vi "PrepLine_window.vi"() -> ()   [LabVIEW 2015]
uses:
  <vilib>/Utility/miscctls.llb/LVPoint32TypeDef.ctl
  global variables.vi
  Classes/StatusLog/StatusLog.lvclass
  Classes/PrepLineObject/PrepLineObject.lvclass
panel:
  out "name of changed":string
  out "Button":u16
  out "Mouse Down \nCoords":T1
  in  "error in (no error)":errorcluster
  out "prepline picture":picture
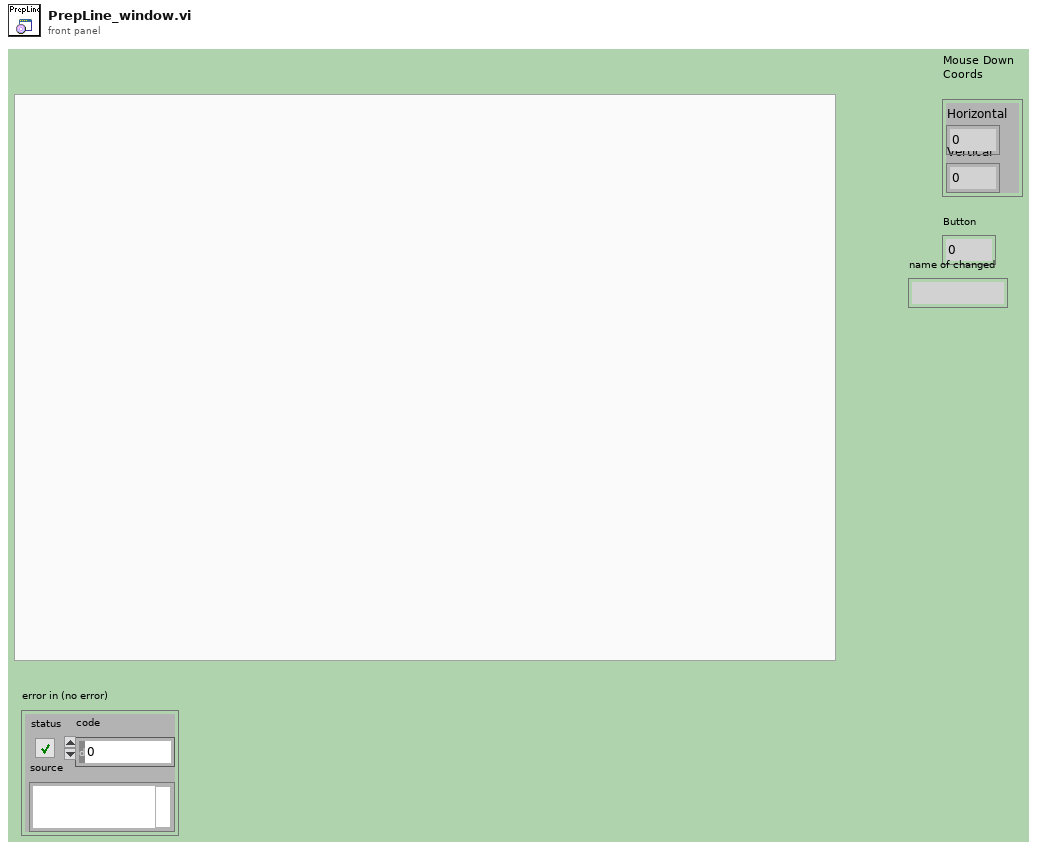
[diagram p1: front panel]
types:
  T1 = typedef "LVPoint32TypeDef.ctl" = cluster{"Horizontal":i32, "Vertical":i32}
  T2 = typedef "LVRectTypeDef.ctl" = cluster{"Left":i16, "Top":i16, "Right":i16, "Bottom":i16}
  T3 = typedef "imagedata.ctl" = cluster{"image type":i32, "image depth":i32, "image":u8[], "mask":u8[], "colors":u32[], "Rectangle":cluster{"left":i16, "top":i16, "right":i16, "bottom":i16}}
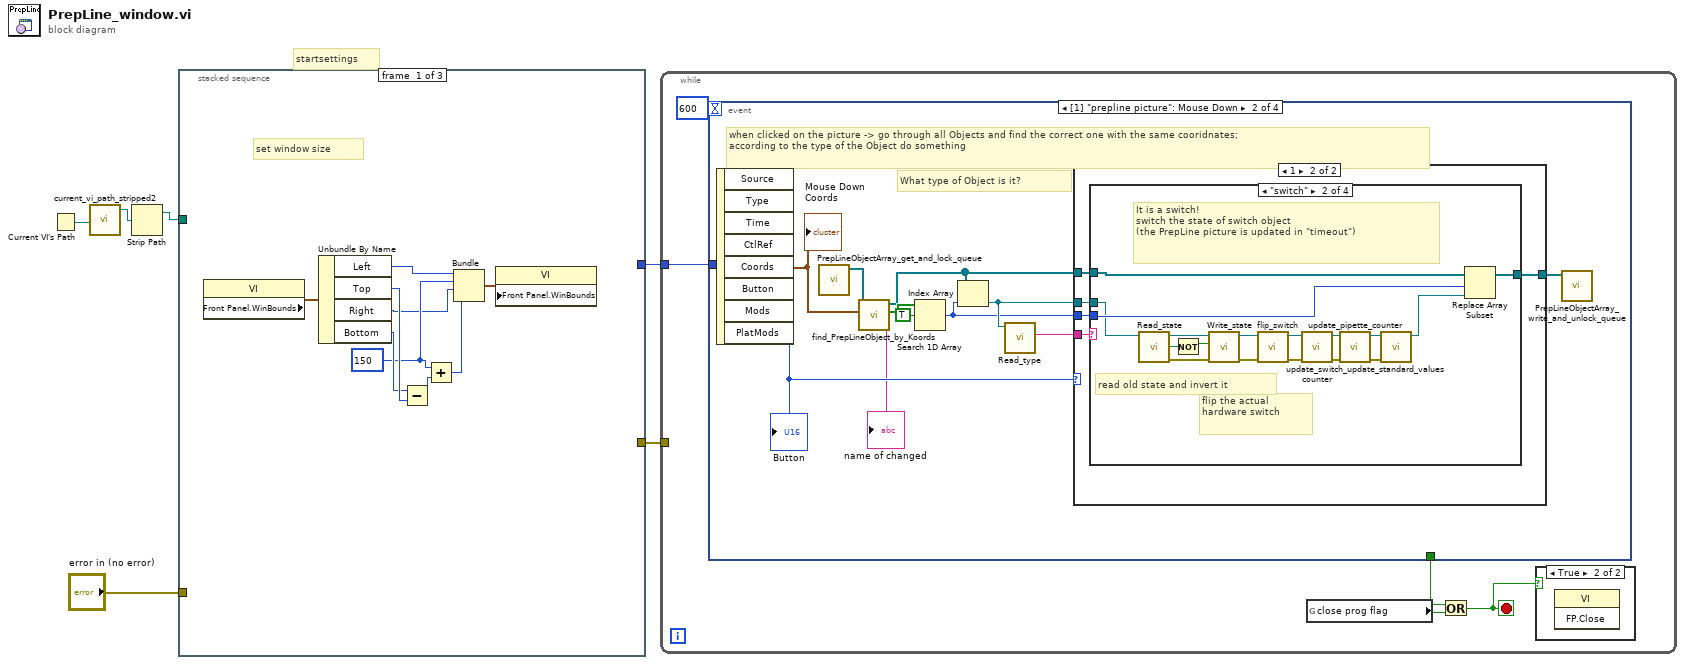
[diagram p0: block diagram]
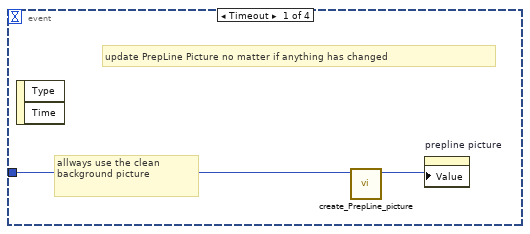
[diagram p3: hidden frame]
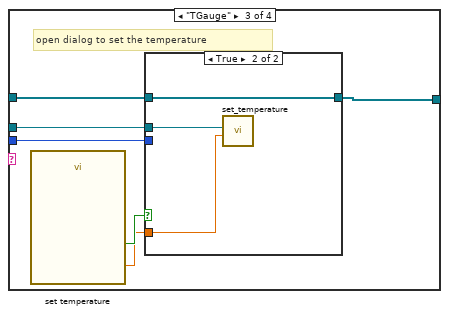
[diagram p6: hidden frame]
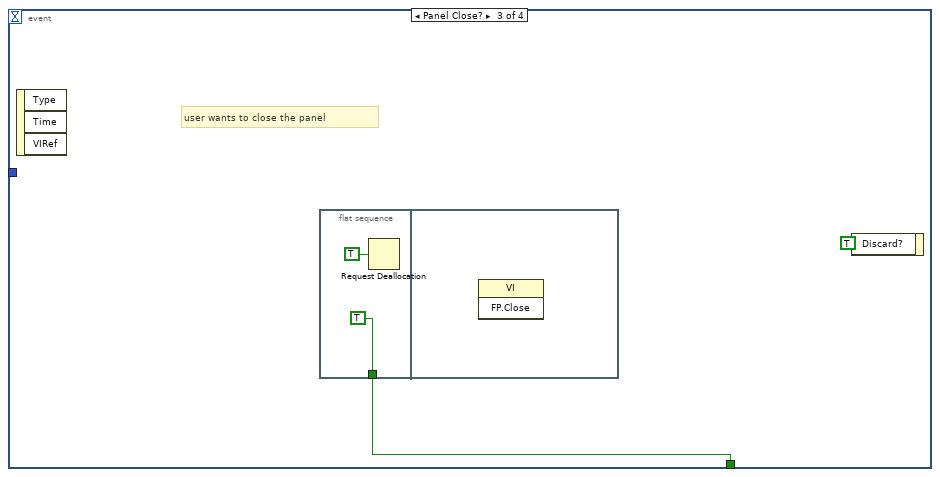
[diagram p9: hidden frame]
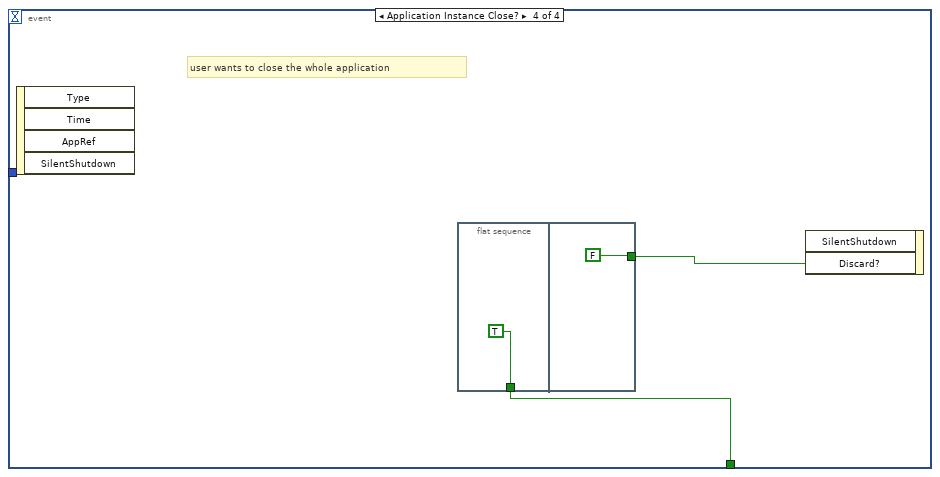
[diagram p10: hidden frame]
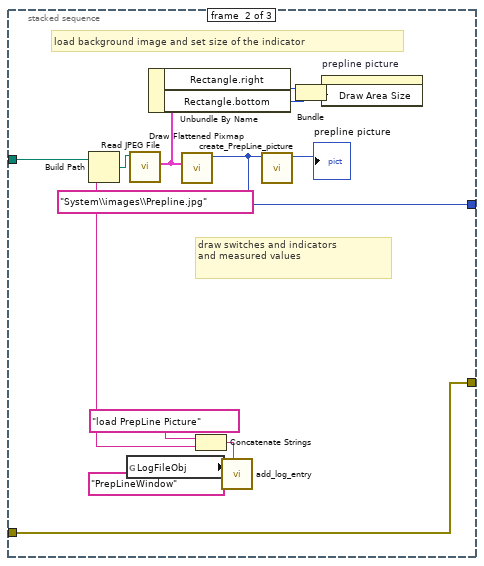
[diagram p11: hidden frame]
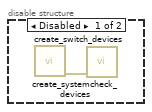
[diagram p13: hidden frame]
diagram:
  # "startsettings"
  n1 = Current VI's Path() -> (path=w3:path)
  n2 = call "current_vi_path_stripped2.vi"("current VI Path"=w3) -> ("current VI Path stripped out"=w1:path)  [unwired: 3 in, 1 out]
  n3 = Strip Path(path=w1) -> (stripped path=w2:path)  [unwired: 1 out]
  n4 = stacked-sequence {
    tunnel: [_ w28 _] -> w6
    tunnel: w2 -> [_ w29 _]
    tunnel: "error in (no error)" -> [_ w28 _]
    tunnel: [_ w16 _] -> w4
    frame #0 {
      w11 = i16 150 ("y")
      # "set window size"
      n5 = property class="VI"() -> ("Front Panel.WinBounds"=w7:T2)  [unwired: 2 in, 2 out]
      n6 = Unbundle By Name(w7) -> ("Left"=w8:i16, "Top"=w15:i16, "Right"=w10:i16, "Bottom"=w14:i16)
      n7 = Subtract(x=w14, y=w15) -> (x-y=w12:i16)
      n8 = Add(x=w11, y=w12) -> (x+y=w13:i16)
      n9 = Bundle("Left"=w8, "y"=w11, "Right"=w10, w13) -> (w9:cluster{"Left":i16, "y":i16, "Right":i16, i16})  [unwired: 1 in]
      n10 = property class="VI"("Front Panel.WinBounds"=w9) -> ()  [unwired: 2 in, 2 out]
    }
    frame #1 {
      w18 = "System\\images\\Prepline.jpg" ("name or relative path")
      # "draw switches and indicators\nand measured values"
      # "load background image and set size of the indicator"
      n11 = Build Path(base path=w29, name or relative path=w18) -> (appended path=w20:path)
      n12 = global read "global variables.vi" "LogFileObj"() -> (w23:refnum<class "StatusLog.lvclass">)
      n13 = call <vilib>:"Read JPEG File.vi"("path to JPEG file"=w20) -> ("image data"=w27:T3)  [unwired: 8 in, 2 out]
      n14 = Unbundle By Name(w27) -> ("Rectangle.right"=w26:i16, "Rectangle.bottom"=w25:i16)
      n15 = call <vilib>:"Draw Flattened Pixmap.vi"("image data"=w27) -> ("new picture"=w16:picture)  [unwired: 8 in]
      n16 = Concatenate Strings("load PrepLine Picture" ("new entry"), w18) -> (w21:string)
      n17 = call-dynamic "add_log_entry.vi"("new entry"=w21, "log identifiers"="PrepLineWindow", "StatusLog in"=w23) -> ()  [unwired: 5 in, 2 out]
      n18 = call "create_PrepLine_picture.vi"("Value in"=w16) -> ("Value out"=→"prepline picture":picture)  [unwired: 10 in]
      n19 = Bundle("right"=w26, "bottom"=w25) -> (w24:cluster{"right":i16, "bottom":i16})  [unwired: 1 in]
      n20 = property on="prepline picture" class="Pict"("Draw Area Size"=w24) -> ()  [unwired: 2 in, 2 out]
    }
    frame #2 {
      # "this is usually done in the main vi of the\nprogram and not here; use thos only\nfor test purposes"
      # "read switch preferences out of switch file\nand generate switch objects - stored together with all\nother objects  in global variable"
      n21 = disable-structure shown="Enabled" {
        frame Disabled {
          n22 = call "create_switch_devices.vi"() -> ("error out"=w30:errorcluster)  [unwired: 11 in]
          n23 = call "create_systemcheck_devices.vi"("error in (no error)"=w30) -> ()  [unwired: 10 in, 1 out]
        }
        frame Enabled {
        }
      }
    }
  }
  n24 = while {
    tunnel: w6 -> [_]
    tunnel: w4 -> [w34]
    stop <- w31 stop-if-true
    n25 = event shown="[1] \"prepline picture\": Mouse Down" {
      selector: _ -> [_ _ _ _]
      dyn-events: _ -> [_ _ _ _]
      timeout: 600 -> [_ _ _ _]
      tunnel: [_ _ w85 w89] -> w33
      tunnel: w34 -> [w36 _ _ _]
      event Timeout {
        # "allways use the clean\nbackground picture"
        # "update PrepLine Picture no matter if anything has changed"
        n26 = event-data() -> ()  [unwired: 1 in, 2 out]
        n27 = call "create_PrepLine_picture.vi"("Value in"=w36) -> ("Value out"=w37:picture)  [unwired: 10 in]
        n28 = property on="prepline picture" class="Pict"("Value"=w37) -> ()  [unwired: 2 in, 2 out]
      }
      event "prepline picture": Mouse Down {
        # "What type of Object is it?"
        # "when clicked on the picture -> go through all Objects and find the correct one with the same cooridnates;\naccording to the type of the Object do something"
        n29 = event-data() -> ("Coords"=w41:T1, "Button"=w44:u16)  [unwired: 1 in, 6 out]
        "Mouse Down \nCoords" <- w41
        "Button" <- w44
        n30 = call "PrepLineObjectArray_get_and_lock_queue.vi"() -> ("PrepLineObjects"=w39:refnum<class "PrepLineObject.lvclass">[])  [unwired: 10 in, 1 out]
        n31 = call "find_PrepLineObject_by_Koords.vi"("Coords"=w41, "PrepLine\nobjects in"=w39) -> ("name of changed"=→"name of changed":string, "changed switch array"=w48:bool[], "PrepLineObjectsOut"=w40:refnum<class "PrepLineObject.lvclass">[])  [unwired: 5 in, 1 out]
        n32 = Search 1D Array(1D array=w48, element=TRUE) -> (index of element=w43:i32)  [unwired: 1 in]
        n33 = Index Array(array=w40, index=w43) -> (element=w46:refnum<class "PrepLineObject.lvclass">)
        n34 = call-dynamic "Read_type.vi"("PrepLinePictureObjects in"=w46) -> ("type"=w45:string)  [unwired: 8 in, 2 out]
        n35 = case shown="1" w44 {
          tunnel: w40 -> [w49 w54]
          tunnel: w43 -> [_ w53]
          tunnel: w46 -> [_ w52]
          tunnel: w45 -> [_ w51]
          tunnel: [w49 w50] -> w38
          frame 0, Default {
          }
          frame 1 {
            n36 = case shown="\"switch\"" w51 {
              tunnel: w54 -> [w55 w72 w76 w83]
              tunnel: w53 -> [_ w71 w74 _]
              tunnel: w52 -> [_ w63 w75 _]
              tunnel: [w55 w64 w73 w83] -> w50
              frame "False", Default {
                # "is not an object to interact with"
              }
              frame "switch" {
                # "flip the actual\nhardware switch"
                # "read old state and invert it"
                # "It is a switch!\nswitch the state of switch object \n(the PrepLine picture is updated in \"timeout\")"
                n37 = call-dynamic "Read_state.vi"("PrepLineObject in"=w63) -> ("error out"=w67:errorcluster, "state"=w70:bool, "PrepLineObject out"=w68:refnum<class "PrepLineObject.lvclass">)  [unwired: 8 in]
                n38 = Not(x=w70) -> (.not. x?=w69:bool)
                n39 = call-dynamic "Write_state.vi"("error in (no error)"=w67, "state"=w69, "PrepLineObject in"=w68) -> ("error out"=w66:errorcluster, "PrepLineObject out"=w65:refnum<class "PrepLineObject.lvclass">)  [unwired: 7 in]
                n40 = call "flip_switch.vi"("PrepLineObject.lvclass"=w65, "error in (no error)"=w66) -> ("PrepLineObject out"=w62:refnum<class "PrepLineObject.lvclass">, "error out"=w61:errorcluster)  [unwired: 7 in]
                n41 = call "update_switch_counter.vi"("PrepLineObject.lvclass"=w62, "error in (no error)"=w61) -> ("PrepLineObject out"=w59:refnum<class "PrepLineObject.lvclass">, "error out"=w60:errorcluster)  [unwired: 7 in]
                n42 = call "update_pipette_counter.vi"("error in (no error)"=w60, "PrepLineObject in"=w59) -> ("error out"=w57:errorcluster, "PrepLineObject out"=w58:refnum<class "PrepLineObject.lvclass">)  [unwired: 8 in]
                n43 = call "update_standard_values.vi"("error in (no error)"=w57, "PrepLineObject in"=w58) -> ("PrepLineObject out"=w56:refnum<class "PrepLineObject.lvclass">)  [unwired: 8 in, 1 out]
                n44 = Replace Array Subset(array=w72, new element=w56, index=w71) -> (w64:refnum<class "PrepLineObject.lvclass">[])
              }
              frame "TGauge" {
                # "open dialog to set the temperature"
                n45 = call "set temperature"() -> ("set temp"=w77:dbl, "OK"=w78:bool)  [unwired: 17 in, 1 out]
                n46 = case shown="True" w78 {
                  tunnel: w77 -> [_ w82]
                  tunnel: w76 -> [w79 w81]
                  tunnel: w75 -> [_ w80]
                  tunnel: w74 -> [_ _]
                  tunnel: [w79 w81] -> w73
                  frame False {
                  }
                  frame True {
                    n47 = call "set_temperature.vi"("PrepLineObject.lvclass"=w80, "temperature"=w82) -> ()  [unwired: 7 in, 2 out]
                  }
                }
              }
              frame "PGauge" {
                # "#ClickToShowPlot\ndisplay the plot data in the status window when\nclicked on the control"
              }
            }
          }
        }
        n48 = call "PrepLineObjectArray_write_and_unlock_queue.vi"("PrepLineObjArray"=w38) -> ()  [unwired: 10 in, 1 out]
      }
      event Panel Close? {
        # "user wants to close the panel"
        n49 = event-data() -> ()  [unwired: 1 in, 3 out]
        n50 = flat-sequence {
          tunnel: [TRUE] -> w85
          frame #0 {
            n51 = Request Deallocation(TRUE ("flag")) -> ()
          }
          frame #1 {
            n52 = invoke class="VI" method="FP.Close"() -> ()  [unwired: 3 in, 3 out]
          }
        }
        n53 = event-data("Discard?"=TRUE) -> ()  [unwired: 1 in, 1 out]
      }
      event Application Instance Close? {
        # "user wants to close the whole application"
        n54 = event-data() -> ()  [unwired: 1 in, 4 out]
        n55 = flat-sequence {
          tunnel: [TRUE] -> w89
          tunnel: [FALSE] -> w88
          frame #0 {
          }
          frame #1 {
          }
        }
        n56 = event-data("Discard?"=w88) -> ()  [unwired: 2 in, 1 out]
      }
    }
    n57 = global read "global variables.vi" "close prog flag"() -> (w32:bool)
    n58 = Or(x=w33, y=w32) -> (x .or. y?=w31:bool)
    n59 = case shown="True" w31 {
      frame False {
      }
      frame True {
        n60 = invoke class="VI" method="FP.Close"() -> ()  [unwired: 3 in, 3 out]
      }
    }
  }
